vi "dvp Vi Get Strobe Delay.vi"(10 "pStrobeDelay":dbl, 11 "handle":u32) -> (2 "pStrobeDelay out":dbl, 3 "function return":u32(ring))   [LabVIEW 2018, in "LabViewDVPCamera.lvlib"]
doc: "LabviewDvp2Api dvpStatus dvpViGetStrobeDelay(dvpHandle handle, double *pStrobeDelay);"
uses:
  LabViewDVPCamera.lvlib
  LabViewDVPCamera/LabViewDVPCamera.dll
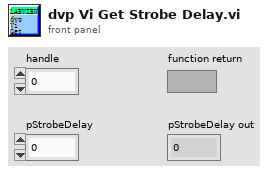
[diagram p1: front panel]
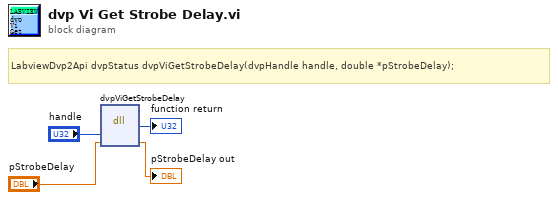
[diagram p0: block diagram]
diagram:
  # "LabviewDvp2Api dvpStatus dvpViGetStrobeDelay(dvpHandle handle, double *pStrobeDelay);"
  n1 = dll-call lib="C:/Program Files (x86)/DVP2 Labview cn 64/Sample/LabViewDVPCamera/LabViewDVPCamera.*" fn="dvpViGetStrobeDelay"("handle"="handle", "pStrobeDelay"="pStrobeDelay") -> (→"function return":u32, "pStrobeDelay"=→"pStrobeDelay out":dbl)  [unwired: 4 in, 2 out]
